vi "ProjectCloseReferences.vi"(11 "error in (no error)":errorcluster) -> (15 "error out":errorcluster)   [LabVIEW 2015, in "ni-veristand-steps-runtime-lib.lvlib"]
uses:
  ni-veristand-steps-runtime-lib.lvlib
  <vilib>/NI Veristand/Execution/AlarmManager/NI_VS AlarmManager ExecutionAPI.lvlib
  <vilib>/NI Veristand/Execution/ChannelFaultManager/NI_VS ChannelFault ExecutionAPI.lvlib
  <vilib>/NI Veristand/Execution/ModelManager/NI_VS ModelManager ExecutionAPI.lvlib
  <vilib>/NI Veristand/Execution/Workspace/NI_VS Workspace ExecutionAPI.lvlib
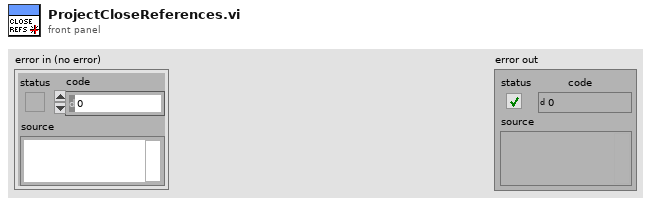
[diagram p1: front panel]
types:
  T1 = typedef "ni-veristand-steps-runtime-lib.lvlib/VeriStand dotNet References.ctl" = cluster{"ModelManager":T2, "AlarmManager":T3, "ChannelFault":T4, "WorkspaceManager":T5, "Project Ref":T6}
  T2 = typedef "NI_VS ModelManager ExecutionAPI.lvlib/ModelManagerAPI.ctl" = refnum<k24>
  T3 = typedef "NI_VS AlarmManager ExecutionAPI.lvlib/AlarmManagerAPI.ctl" = refnum<k24>
  T4 = typedef "NI_VS ChannelFault ExecutionAPI.lvlib/ChannelFaultAPI.ctl" = refnum<k24>
  T5 = typedef "NI_VS Workspace ExecutionAPI.lvlib/WorkspaceAPI.ctl" = refnum<k24>
  T6 = typedef "NI_VS Project ExecutionAPI.lvlib/Project Ref.ctl" = refnum<k24>
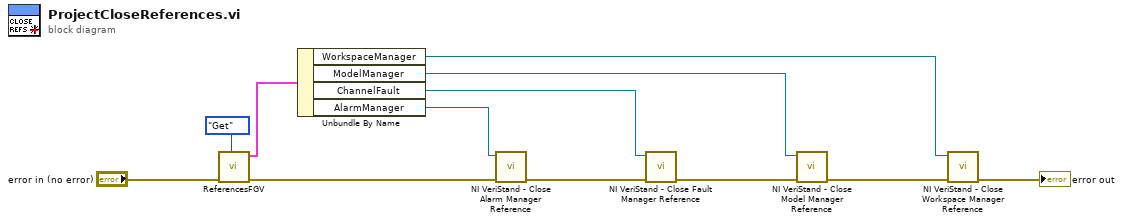
[diagram p0: block diagram]
diagram:
  n1 = call "ReferencesFGV.vi"("Get/Set"=enum16{"Get", "Set"}."Get", "error in (no error)"="error in (no error)") -> ("error out"=w9:errorcluster, "VeriStand dotNET Refs out"=w10:T1)  [unwired: 8 in]
  n2 = Unbundle By Name(w10) -> ("WorkspaceManager"=w1:T5, "ModelManager"=w2:T2, "ChannelFault"=w3:T4, "AlarmManager"=w4:T3)
  n3 = call <vilib>:"NI VeriStand - Close Alarm Manager Reference.vi"("error in (no error)"=w9, "AlarmManager"=w4) -> ("error out"=w8:errorcluster)  [unwired: 9 in]
  n4 = call <vilib>:"NI VeriStand - Close Fault Manager Reference.vi"("error in (no error)"=w8, "ChannelFault"=w3) -> ("error out"=w7:errorcluster)  [unwired: 9 in]
  n5 = call <vilib>:"NI VeriStand - Close Model Manager Reference.vi"("error in (no error)"=w7, "ModelManager"=w2) -> ("error out"=w6:errorcluster)  [unwired: 9 in]
  n6 = call <vilib>:"NI VeriStand - Close Workspace Manager Reference.vi"("error in (no error)"=w6, "WorkspaceManager"=w1) -> ("error out"=→"error out":errorcluster)  [unwired: 9 in]
